vi "tcp_client_many.vi"() -> ()   [LabVIEW 2019]
panel:
  out "spill_id 10":i32
  out "status 10":bool=TRUE
  out "count 10":i32
  out "spill_id 9":i32
  out "status 9":bool=TRUE
  out "count 9":i32
  out "spill_id 8":i32
  out "status 8":bool=TRUE
  out "count 8":i32
  out "spill_id 7":i32
  out "status 7":bool=TRUE
  out "count 7":i32
  out "spill_id 6":i32
  out "status 6":bool=TRUE
  out "count 6":i32
  out "spill_id 5":i32
  out "status 5":bool=TRUE
  out "count 5":i32
  out "spill_id 4":i32
  out "status 4":bool=TRUE
  out "count 4":i32
  out "spill_id 3":i32
  out "status 3":bool=TRUE
  out "count 3":i32
  out "spill_id 2":i32
  out "status 2":bool=TRUE
  out "count 2":i32
  out "count":i32
  out "status":bool=TRUE
  out "spill_id":i32
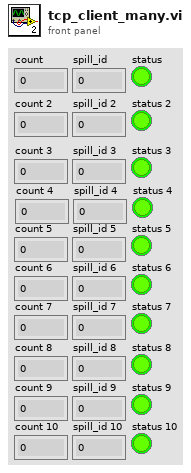
[diagram p1: front panel]
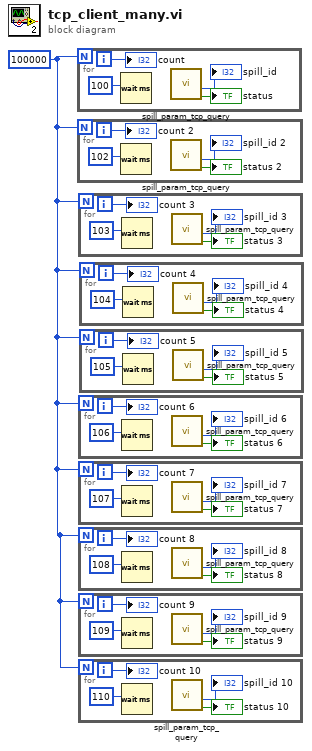
[diagram p0: block diagram]
diagram:
  w1 = 100000
  n1 = for "TCP/IP Query Client" {
    N: w1 -> [_]
    i -> [w2]
    n2 = Wait (ms)(milliseconds to wait=u32 100) -> ()  [unwired: 1 out]
    n3 = call "spill_param_tcp_query.vi"() -> ("status"=→"status":bool, "spill_id"=→"spill_id":i32)  [unwired: 6 in, 2 out]
    "count" <- w2
  }
  n4 = for "TCP/IP Query Client" {
    N: w1 -> [_]
    i -> [w6]
    n5 = Wait (ms)(milliseconds to wait=u32 102) -> ()  [unwired: 1 out]
    n6 = call "spill_param_tcp_query.vi"() -> ("status"=→"status 2":bool, "spill_id"=→"spill_id 2":i32)  [unwired: 6 in, 2 out]
    "count 2" <- w6
  }
  n7 = for "TCP/IP Query Client" {
    N: w1 -> [_]
    i -> [w10]
    n8 = Wait (ms)(milliseconds to wait=u32 103) -> ()  [unwired: 1 out]
    n9 = call "spill_param_tcp_query.vi"() -> ("status"=→"status 3":bool, "spill_id"=→"spill_id 3":i32)  [unwired: 6 in, 2 out]
    "count 3" <- w10
  }
  n10 = for "TCP/IP Query Client" {
    N: w1 -> [_]
    i -> [w14]
    n11 = Wait (ms)(milliseconds to wait=u32 106) -> ()  [unwired: 1 out]
    n12 = call "spill_param_tcp_query.vi"() -> ("status"=→"status 6":bool, "spill_id"=→"spill_id 6":i32)  [unwired: 6 in, 2 out]
    "count 6" <- w14
  }
  n13 = for "TCP/IP Query Client" {
    N: w1 -> [_]
    i -> [w18]
    n14 = Wait (ms)(milliseconds to wait=u32 107) -> ()  [unwired: 1 out]
    n15 = call "spill_param_tcp_query.vi"() -> ("status"=→"status 7":bool, "spill_id"=→"spill_id 7":i32)  [unwired: 6 in, 2 out]
    "count 7" <- w18
  }
  n16 = for "TCP/IP Query Client" {
    N: w1 -> [_]
    i -> [w22]
    n17 = Wait (ms)(milliseconds to wait=u32 108) -> ()  [unwired: 1 out]
    n18 = call "spill_param_tcp_query.vi"() -> ("status"=→"status 8":bool, "spill_id"=→"spill_id 8":i32)  [unwired: 6 in, 2 out]
    "count 8" <- w22
  }
  n19 = for "TCP/IP Query Client" {
    N: w1 -> [_]
    i -> [w26]
    n20 = Wait (ms)(milliseconds to wait=u32 109) -> ()  [unwired: 1 out]
    n21 = call "spill_param_tcp_query.vi"() -> ("status"=→"status 9":bool, "spill_id"=→"spill_id 9":i32)  [unwired: 6 in, 2 out]
    "count 9" <- w26
  }
  n22 = for "TCP/IP Query Client" {
    N: w1 -> [_]
    i -> [w30]
    n23 = Wait (ms)(milliseconds to wait=u32 110) -> ()  [unwired: 1 out]
    n24 = call "spill_param_tcp_query.vi"() -> ("status"=→"status 10":bool, "spill_id"=→"spill_id 10":i32)  [unwired: 6 in, 2 out]
    "count 10" <- w30
  }
  n25 = for "TCP/IP Query Client" {
    N: w1 -> [_]
    i -> [w34]
    n26 = Wait (ms)(milliseconds to wait=u32 104) -> ()  [unwired: 1 out]
    n27 = call "spill_param_tcp_query.vi"() -> ("status"=→"status 4":bool, "spill_id"=→"spill_id 4":i32)  [unwired: 6 in, 2 out]
    "count 4" <- w34
  }
  n28 = for "TCP/IP Query Client" {
    N: w1 -> [_]
    i -> [w38]
    n29 = Wait (ms)(milliseconds to wait=u32 105) -> ()  [unwired: 1 out]
    n30 = call "spill_param_tcp_query.vi"() -> ("status"=→"status 5":bool, "spill_id"=→"spill_id 5":i32)  [unwired: 6 in, 2 out]
    "count 5" <- w38
  }
